vi "modem2.vi"() -> ()   [LabVIEW 2010]
uses:
  My Application/data/user32.dll
panel:
  out "error out":errorcluster
  out "String":string
  out "modem used":bool
  out "Boolean":bool caption="цикл"
  in  "stop":bool
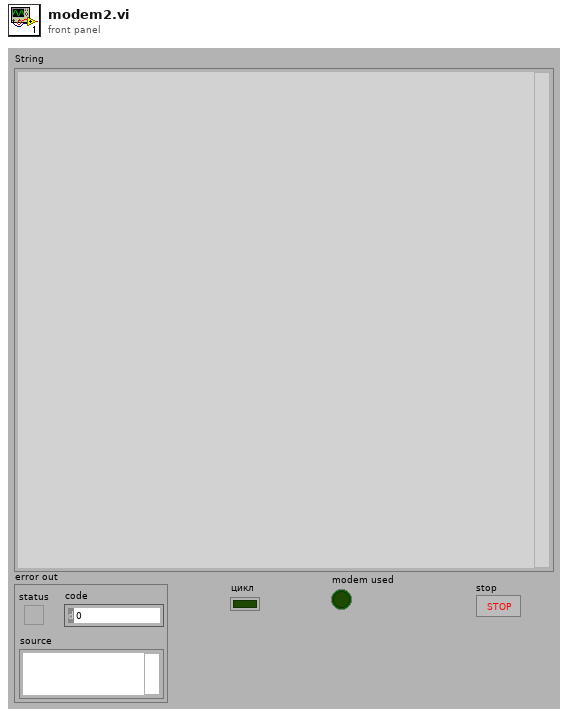
[diagram p1: front panel]
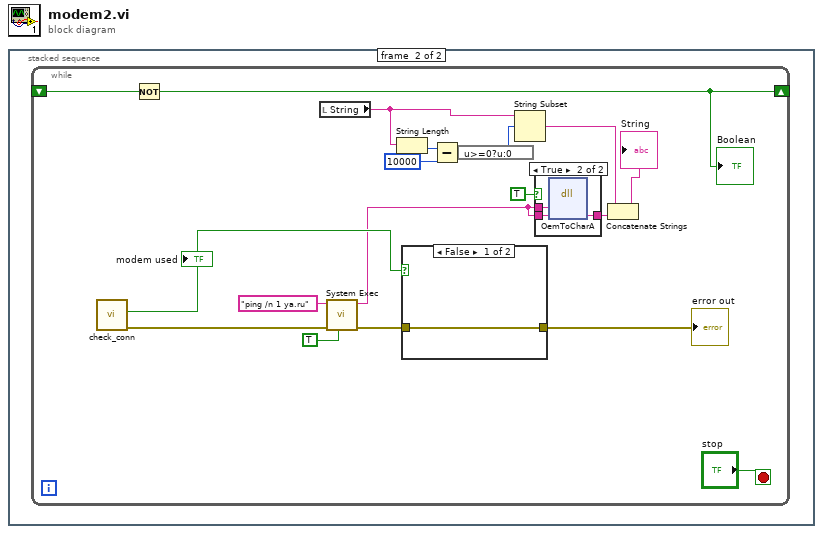
[diagram p0: block diagram]
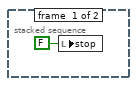
[diagram p2: hidden frame]
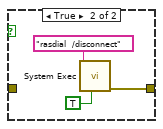
[diagram p4: hidden frame]
diagram:
  n1 = stacked-sequence {
    frame #0 {
      n2 = local write "stop"(FALSE ("stop")) -> ()
    }
    frame #1 {
      n3 = while {
        shift-right: [w18] -> _
        shift-left: _ -> [w19]
        stop <- "stop" stop-if-true
        n4 = call "check_conn.vi"() -> ("error out"=w17:errorcluster, "modem used"=w13:bool)  [unwired: 6 in]
        "modem used" <- w13
        n5 = Not(x=w19) -> (.not. x?=w18:bool)
        "Boolean" <- w18
        n6 = local read "String"() -> (w10:string)
        n7 = call <vilib>:"System Exec.vi"("run minimized? (F)"=TRUE, "error in (no error)"=w17, "command line"="ping /n 1 ya.ru") -> ("error out"=w14:errorcluster, "standard output"=w2:string)  [unwired: 5 in, 2 out]
        n8 = String Length(string=w10) -> (length=w9:i32)
        n9 = case shown="False" w13 {
          tunnel: w14 -> [w25 _]
          tunnel: [w25 w26] -> w5
          frame False {
          }
          frame True {
            n10 = call <vilib>:"System Exec.vi"("run minimized? (F)"=TRUE, "command line"="rasdial  /disconnect") -> ("error out"=w26:errorcluster)  [unwired: 6 in, 3 out]
          }
        }
        "error out" <- w5
        n11 = Subtract(x=w9, y=10000) -> (x-y=w8:i32)
        n12 = expression code="u>=0?u:0"(w8) -> (w6:i32)
        n13 = String Subset(string=w10, offset (0)=w6) -> (substring=w12:string)  [unwired: 1 in]
        n14 = case shown="True" TRUE {
          tunnel: [w21 w24] -> w4
          tunnel: w2 -> [w21 w23]
          tunnel: w2 -> [_ w22]
          frame False {
          }
          frame True {
            n15 = dll-call lib="C:/skill/My Application/data/user32.dll" fn="OemToCharA"("src"=w23, "dst"=w22) -> ("dst"=w24:string)  [unwired: 5 in, 2 out]
          }
        }
        n16 = Concatenate Strings(w12, w4) -> (→"String":string)
      }
    }
  }
